vi "MES_PATH_SET.vi"() -> ()   [LabVIEW 2018]
uses:
  Global.vi
  <vilib>/Utility/config.llb/Write Key (String).vi
  <vilib>/Utility/config.llb/Read Key (String).vi
  <vilib>/Utility/config.llb/NI_LVConfig.lvlib
panel:
  in  "字符串":string
  in  "路径:":path
  in  "Save":bool
  in  "Quit":bool
  out "value":string caption="值"
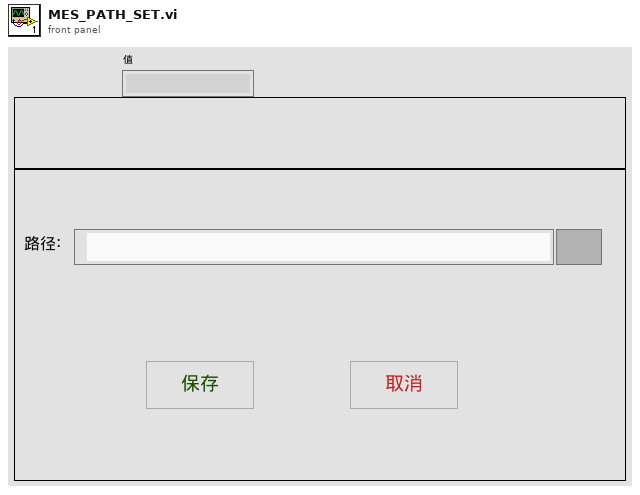
[diagram p1: front panel]
types:
  T1 = typedef "NI_LVConfig.lvlib/Config Data RefNum.ctl" = refnum<k1>
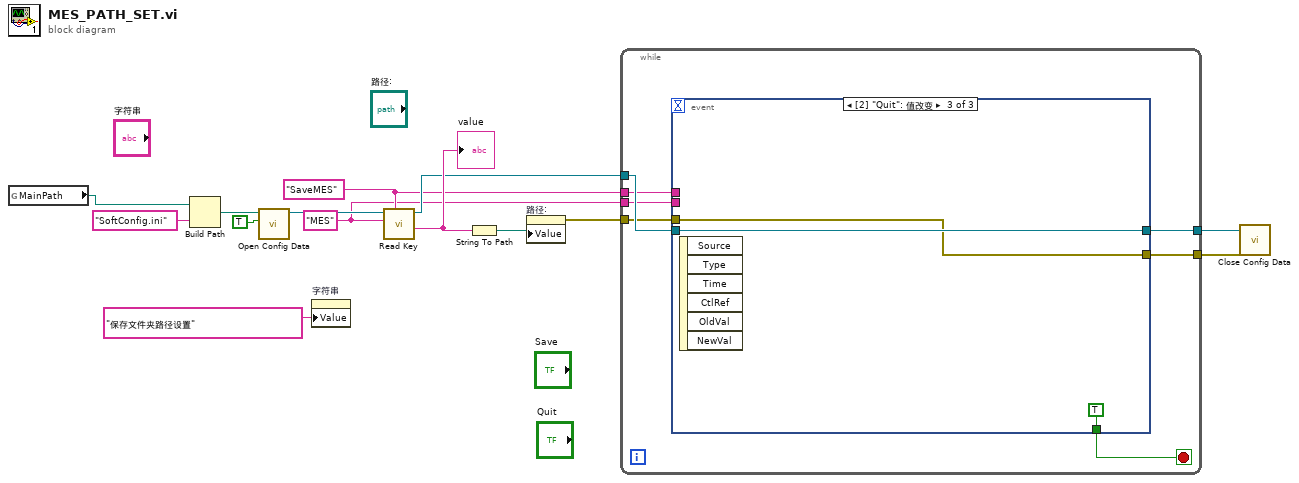
[diagram p0: block diagram]
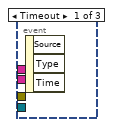
[diagram p2: hidden frame]
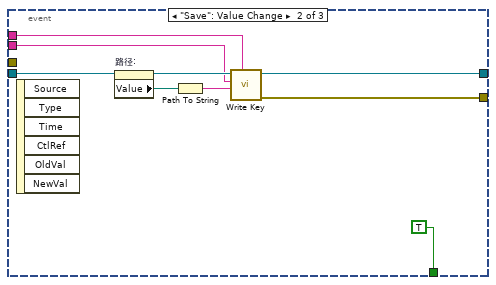
[diagram p3: hidden frame]
diagram:
  w4 = "MES" ("key")
  w5 = "SaveMES"
  n1 = global read "Global.vi" "MainPath"() -> (w13:path)
  n2 = Build Path(base path=w13, name or relative path="SoftConfig.ini" ("名称或相对路径")) -> (appended path=w11:path)
  n3 = call <vilib>:"Open Config Data.vi"("create file if necessary (T)"=TRUE, "configuration file path"=w11) -> ("refnum"=w14:T1)  [unwired: 7 in, 2 out]
  n4 = property on="字符串" class="Str"("Value"="保存文件夹路径设置" ("字符串")) -> ()  [unwired: 2 in, 2 out]
  n5 = call-poly <vilib>:"Read Key.vi"("section"=w5, "key"=w4, "refnum"=w14) -> ("value"=w8:string, "refnum out"=w6:T1)  [unwired: 5 in, 2 out]
  "value" <- w8
  n6 = String To Path(string=w8) -> (path=w7:path)
  n7 = property on="路径:" class="Path"("Value"=w7) -> (error out=w1:errorcluster)  [unwired: 2 in, 1 out]
  n8 = while {
    tunnel: w6 -> [w21]
    tunnel: w5 -> [w20]
    tunnel: w4 -> [w19]
    tunnel: [w18] -> w3
    tunnel: [w17] -> w2
    tunnel: w1 -> [w15]
    stop <- w16 stop-if-true
    n9 = event shown="[2] \"Quit\": 值改变" {
      selector: _ -> [_ _ _]
      dyn-events: _ -> [_ _ _]
      timeout: _ -> [_ _ _]
      tunnel: w21 -> [_ w29 w31]
      tunnel: w20 -> [_ w28 _]
      tunnel: w19 -> [_ w27 _]
      tunnel: [_ w24 w31] -> w18
      tunnel: [_ w23 w30] -> w17
      tunnel: [_ TRUE TRUE] -> w16
      tunnel: w15 -> [_ _ w30]
      event Timeout {
        n10 = event-data() -> ()  [unwired: 1 in, 3 out]
      }
      event "Save": Value Change {
        n11 = event-data() -> ()  [unwired: 1 in, 6 out]
        n12 = property on="路径:" class="Path"() -> ("Value"=w25:path)  [unwired: 2 in, 2 out]
        n13 = Path To String(path=w25) -> (string=w26:string)
        n14 = call-poly <vilib>:"Write Key.vi"("section"=w28, "value"=w26, "key"=w27, "refnum"=w29) -> ("error out"=w23:errorcluster, "refnum out"=w24:T1)  [unwired: 5 in, 1 out]
      }
      event "Quit": Value Change {
        n15 = event-data() -> ()  [unwired: 1 in, 6 out]
      }
    }
  }
  n16 = call <vilib>:"Close Config Data.vi"("error in (no error)"=w2, "refnum"=w3) -> ()  [unwired: 8 in, 2 out]
